vi "AlliGator Get Time Stamps & Settings from .set File.vi"(8 "Error In":errorcluster, 9 ".set File Names":string[](array[string]), 11 "Folder Path":path) -> (0 "Error Out":errorcluster, 1 "Time Stamps":dbl[](array[numeric]), 3 "Settings String":string)   [LabVIEW 2021, in "AlliGator Files.lvlib"]
doc: "Tries to extract FLI dataset metadata corresponding to one of LaVision formats."
uses:
  AlliGator Files.lvlib
  Time/PicoStart Date.ctl
  Time/Time.lvlib
  Strings/Strings.lvlib
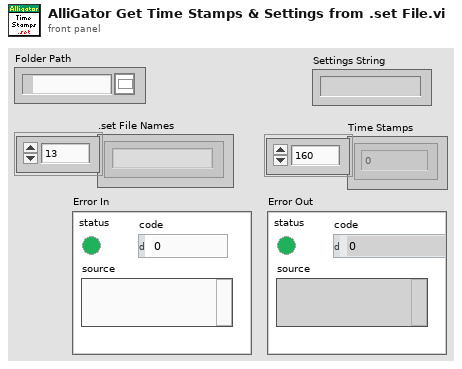
[diagram p1: front panel]
types:
  T1 = typedef "Time.lvlib/PicoStart Date.ctl" = cluster{"Day in Week":string, "Month":string, "Day":i32, "Hours":i32, "Minutes":i32, "Seconds":i32, "Year":i32}
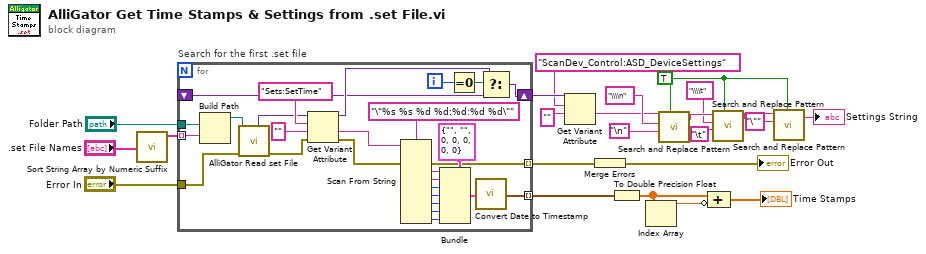
[diagram p0: block diagram]
diagram:
  w17 = TRUE ("replace all? (F)")
  n1 = call "Sort String Array by Numeric Suffix.vi"("String Array"=".set File Names") -> ("Sorted String Array"=w21:string[])  [unwired: 8 in, 2 out]
  n2 = for "Search for the first .set file" {
    tunnel: w21 -> [w49] mode=indexing
    tunnel: "Folder Path" -> [w50]
    tunnel: [w47] -> w20 mode=indexing
    shift-right: [w30] -> w22
    shift-left: _ -> [w29]
    tunnel: "Error In" -> [w28]
    tunnel: [w25] -> w2 mode=indexing
    i -> [w33]
    n3 = Build Path(base path=w50, name or relative path=w49) -> (appended path=w48:path)
    n4 = call "AlliGator Read set File.vi"("Error In"=w28, "Image Folder Path"=w48) -> ("Error Out"=w27:errorcluster, "File info"=w24:variant)  [unwired: 5 in, 3 out]
    n5 = Get Variant Attribute(Variant=w24, name="Sets:SetTime", default value (empty Variant)="" ("name"), error in=w27) -> (duplicate Variant=w31:variant, value=w44:string, error out=w26:errorcluster)  [unwired: 1 out]
    n6 = Scan From String(format string="\"%s %s %d %d:%d:%d %d\"", input string=w44, error in=w26) -> (error out=w25:errorcluster, output 1=w42:string, output 2=w41:string, output 3=w40:i32, output 4=w39:i32, output 5=w38:i32, output 6=w37:i32, output 7=w36:i32)  [unwired: 8 in, 2 out]
    n7 = Bundle(cluster=T1 {"Day in Week"="", "Month"="", "Day"=0, "Hours"=0, "Minutes"=0, "Seconds"=0, "Year"=0}, "Day in Week"=w42, "Month"=w41, "Day"=w40, "Hours"=w39, "Minutes"=w38, "Seconds"=w37, "Year"=w36) -> (w35:T1)
    n8 = Equal To 0?(x=w33) -> (x = 0?=w32:bool)
    n9 = call "Convert Date to Timestamp.vi"("Date"=w35) -> ("Time Stamp"=w47:timestamp)  [unwired: 8 in]
    n10 = Select(t=w31, s=w32, f=w29) -> (s? t:f=w30:variant)
  }
  n11 = Get Variant Attribute(Variant=w22, name="ScanDev_Control:ASD_DeviceSettings", default value (empty Variant)="" ("name")) -> (value=w11:string)  [unwired: 1 in, 3 out]
  n12 = Merge Errors(w2) -> (→"Error Out":errorcluster)
  n13 = To Double Precision Float(number=w20) -> (double precision float=w6:dbl[])
  n14 = Index Array(array=w6) -> (element=w4:dbl)  [unwired: 1 in]
  n15 = call <vilib>:"Search and Replace Pattern.vi"("string"=w11, "regular expression (\"\")"="\\\\n" ("regular expression (\"\")"), "replace string (\"\")"="\n", "replace all? (F)"=w17) -> ("result string"=w14:string)  [unwired: 1 in, 1 out]
  n16 = Compound Arithmetic op=ADD(w6, invert w4) -> (→"Time Stamps":dbl[])
  n17 = call <vilib>:"Search and Replace Pattern.vi"("string"=w14, "regular expression (\"\")"="\\\\t" ("regular expression (\"\")"), "replace string (\"\")"="\t", "replace all? (F)"=w17) -> ("result string"=w16:string)  [unwired: 1 in, 1 out]
  n18 = call <vilib>:"Search and Replace Pattern.vi"("string"=w16, "regular expression (\"\")"="\"" ("regular expression (\"\")"), "replace all? (F)"=w17) -> ("result string"=→"Settings String":string)  [unwired: 2 in, 1 out]
